vi "ReadEprom.vi"() -> ()   [LabVIEW 2017]
uses:
  Traverse/ICNC/ICNC2.lvlib
panel:
  out "number":i32
  in  "Numeric 2":i32=1
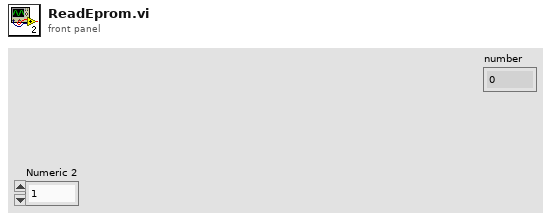
[diagram p1: front panel]
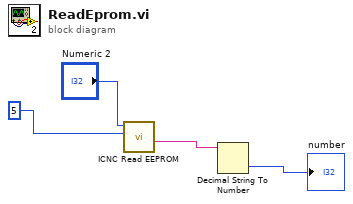
[diagram p0: block diagram]
diagram:
  n1 = call <menus>:"ICNC Read EEPROM.vi"("Length"=5, "StartAdress"="Numeric 2") -> ("Value out"=w2:string)  [unwired: 7 in, 2 out]
  n2 = Decimal String To Number(string=w2) -> (number=→"number":i32)  [unwired: 2 in, 1 out]
